vi "Process Data.vi"(8 "error in (no error)":errorcluster, 9 "Channel Data":T3 {"Current Values"."State" items=["Channel is stopped", "Channel is running", "Channel is paused"]; "Current Values"."I Range" items=["I range 100 pA SP-300 series", "I range 1 nA VMP3 / SP-300 series", "I range 10 nA VMP3 / SP-300 series", "I range 100 nA VMP3 / SP-300 series", "I range 1 uA VMP3 / SP-300 series", "I range 10 uA VMP3 / SP-300 series", "I range 100 uA VMP3 / SP-300 series", "I range 1 mA VMP3 / SP-300 series", "I range 10 mA VMP3 / SP-300 series", "I range 100 mA VMP3 / SP-300 series", "I range 1 A VMP3 / SP-300 series", "Booster VMP3 / SP-300 series", "Auto range VMP3 / SP-300 series"]; "Current Values"."Hardware Option Error Code" items=["No Error"=0, "no instrument connected"=-1, "connection in progress"=-2, "selected channel(s) unplugged"=-3, "invalid function parameters"=-4, "selected file does not exist"=-5, "function failed"=-6, "no channel selected"=-7, "invalid instrument configuration"=-8, "EC-Lab firmware loaded on the instrument"=-9, "library not correctly loaded in memory"=-10, "USB library not correctly loaded in memory"=-11, "function of the library already in progress"=-12, "selected channel(s) already used"=-13, "device not allowed"=-14, "Invalid update function parameters"=-15, "internal instrument communication failed"=-101, "too many data to transfer from the instrument (device error)"=-102, "selected channel(s) unplugged (device error)"=-103, "instrument response error"=-104, "invalid message size"=-105]}, 11 "Potentiostat Galvanostat in":refnum<class "Potentiostat Galvanostat.lvclass">) -> (0 "error out":errorcluster, 1 "Processed Data":T1, 2 "Column Names":T2, 3 "Potentiostat Galvanostat out":refnum<class "Potentiostat Galvanostat.lvclass">)   [LabVIEW 2018, in "Potentiostat Galvanostat.lvclass"]
uses:
  Potentiostat Galvanostat.lvclass
  Controls/Channel Data.ctl
  Controls/Process Data.ctl
  Controls/Data Information.ctl
  Controls/Technique ID.ctl
  Controls/Current Values.ctl
  Controls/Channel State.ctl
  Controls/Current Range.ctl
  Controls/Error Codes.ctl
  Controls/Processed Data Column Names.ctl
  Controls/Processed Data.ctl
  Potentiostat Galvanostat.lvclass/Potentiostat Galvanostat.ctl
  Controls/OCV Processed Data Columns.ctl
  Controls/CA-CP Processed Data Columns.ctl
  Controls/CV Processed Data Columns.ctl
  Controls/PEIS-GEIS P0 Processed Data Columns.ctl
  Controls/PEIS-GEIS P1 Processed Data Columns.ctl
  BL_GetErrorMsg.vi
  <vilib>/Utility/error.llb/Error Cluster From Error Code.vi
  <vilib>/Utility/Data Type/NI_Data Type.lvlib
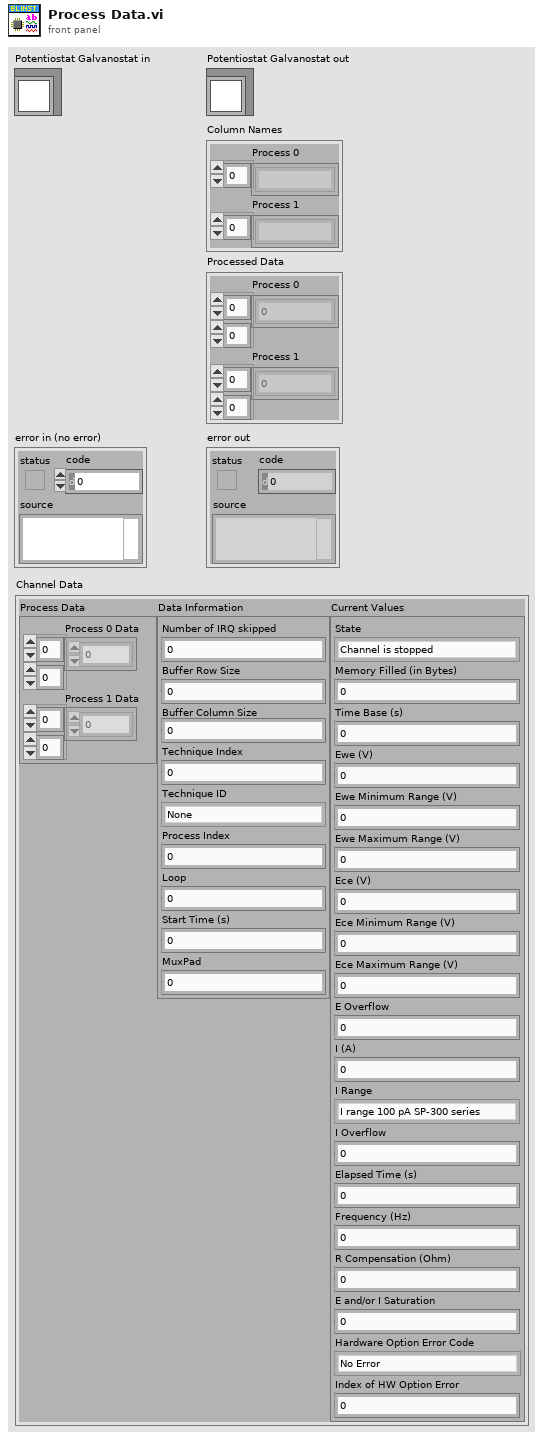
[diagram p1: front panel]
types:
  T1 = typedef "Potentiostat Galvanostat.lvclass/Processed Data.ctl" = cluster{"Process 0":dbl[][], "Process 1":dbl[][]}
  T2 = typedef "Potentiostat Galvanostat.lvclass/Processed Data Column Names.ctl" = cluster{"Process 0":string[], "Process 1":string[]}
  T3 = typedef "Potentiostat Galvanostat.lvclass/Channel Data.ctl" = cluster{"Process Data":T4, "Data Information":T5, "Current Values":T7}
  T4 = typedef "Potentiostat Galvanostat.lvclass/Process Data.ctl" = cluster{"Process 0 Data":sgl[][], "Process 1 Data":sgl[][]}
  T5 = typedef "Potentiostat Galvanostat.lvclass/Data Information.ctl" = cluster{"Number of IRQ skipped":i32, "Buffer Row Size":i32, "Buffer Column Size":i32, "Technique Index":i32, "Technique ID":T6, "Process Index":i32, "Loop":i32, "Start Time (s)":sgl, "MuxPad":i32}
  T6 = typedef "Potentiostat Galvanostat.lvclass/Technique ID.ctl" = i32
  T7 = typedef "Potentiostat Galvanostat.lvclass/Current Values.ctl" = cluster{"State":T8, "Memory Filled (in Bytes)":i32, "Time Base (s)":sgl, "Ewe (V)":sgl, "Ewe Minimum Range (V)":sgl, "Ewe Maximum Range (V)":sgl, "Ece (V)":sgl, "Ece Minimum Range (V)":sgl, "Ece Maximum Range (V)":sgl, "E Overflow":i32, "I (A)":sgl, "I Range":T9, "I Overflow":i32, "Elapsed Time (s)":dbl, "Frequency (Hz)":sgl, "R Compensation (Ohm)":sgl, "E and/or I Saturation":sgl, "Hardware Option Error Code":T10, "Index of HW Option Error":i32}
  T8 = typedef "Potentiostat Galvanostat.lvclass/Channel State.ctl" = i32
  T9 = typedef "Potentiostat Galvanostat.lvclass/Current Range.ctl" = i32
  T10 = typedef "Potentiostat Galvanostat.lvclass/Error Codes.ctl" = i32
  T11 = typedef "Potentiostat Galvanostat.lvclass/OCV Processed Data Columns.ctl" = enum16{"Time /s", "Ewe /V", "Ece /V"}
  T12 = typedef "Potentiostat Galvanostat.lvclass/CA-CP Processed Data Columns.ctl" = enum16{"Time /s", "Ewe /V", "I /A", "Cycle", "Q /C", "log(| I /A |)", "Power /W", "| Power /W |"}
  T13 = typedef "Potentiostat Galvanostat.lvclass/CV Processed Data Columns.ctl" = enum16{"Time /s", "Ece /V", "I /A", "Ewe /V", "Cycle", "Q /C", "log(| I /A |)", "Power /W", "| Power /W |"}
  T14 = typedef "Potentiostat Galvanostat.lvclass/PEIS-GEIS P0 Processed Data Columns.ctl" = enum16{"Time /s", "Ewe /V", "Iwe /A"}
  T15 = typedef "Potentiostat Galvanostat.lvclass/PEIS-GEIS P1 Processed Data Columns.ctl" = enum16{"Frequency /Hz", "| Ewe /V |", "| Iwe /A |", "Phase(Zwe) /rad", "Ewe /V", "Iwe /A", "Ewe Range", "| Ece /V |", "| Ice /A |", "Phase(Zce) /rad", "Ece /V", "Ice /A", "Ece Range", "Time /s", "I Range", "log(| Frequuency /Hz |)", "log(| Iwe /A |)", "log(| Ice /A  |)", "Phase(Zwe) /deg", "Phase(Zce) /deg", "Zwe /ohms", "Zce /ohms", "log(| Zwe /Ohms |)", "log(| Zce /Ohms |)", "-Im(Zwe) ", "-Im(Zce)", "Re(Zwe)", "Re(Zce)"}
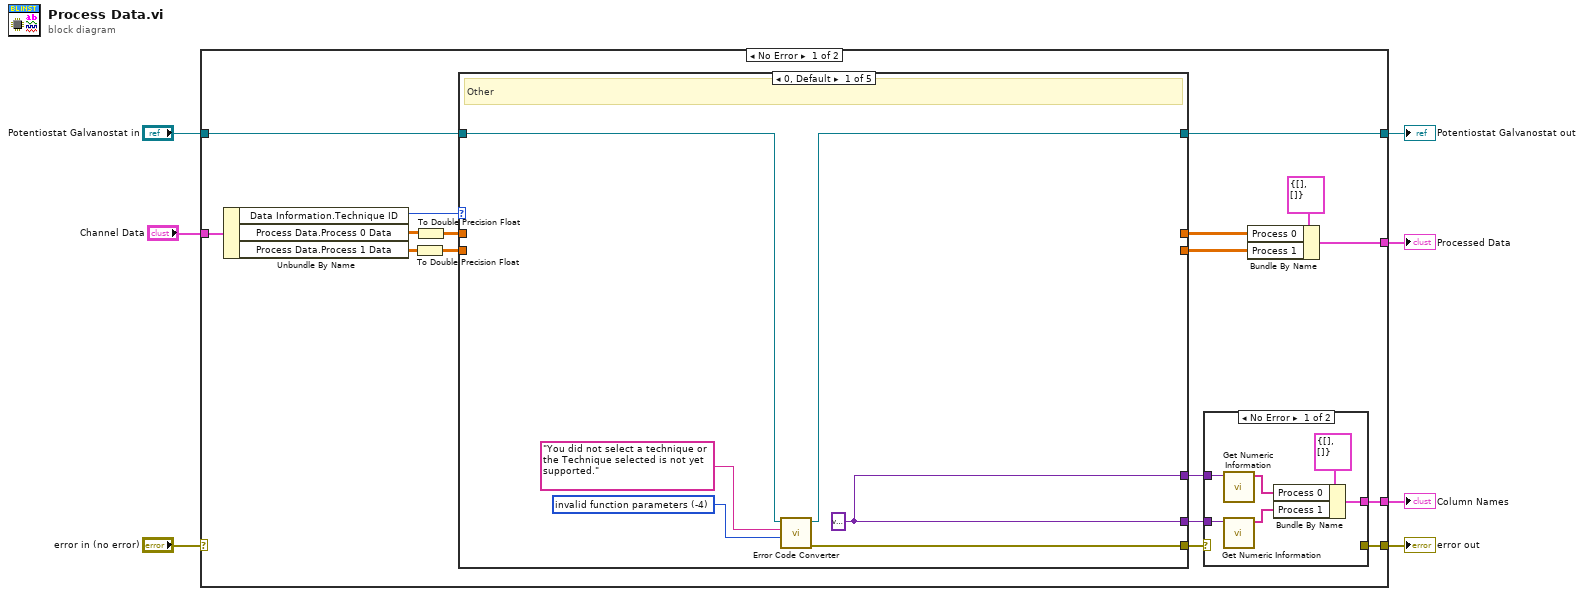
[diagram p0: block diagram]
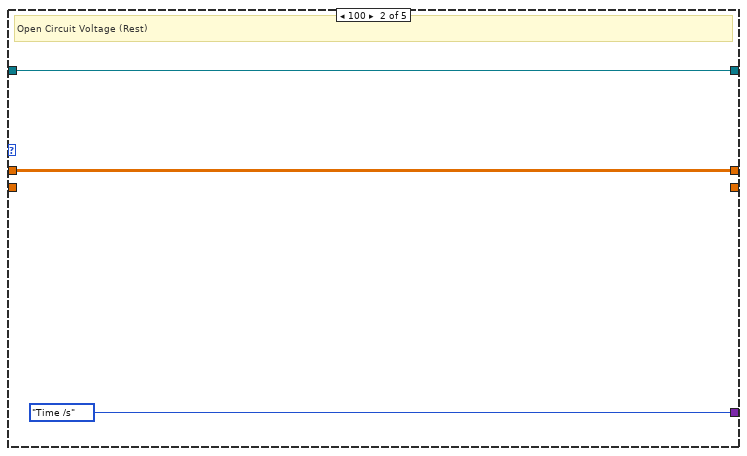
[diagram p3: hidden frame]
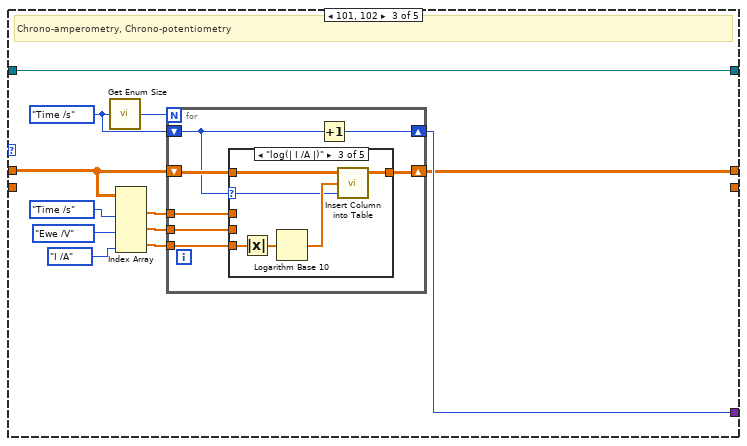
[diagram p4: hidden frame]
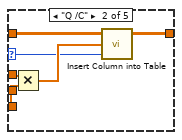
[diagram p6: hidden frame]
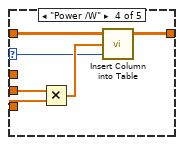
[diagram p7: hidden frame]
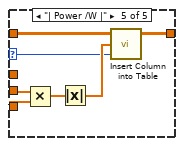
[diagram p8: hidden frame]
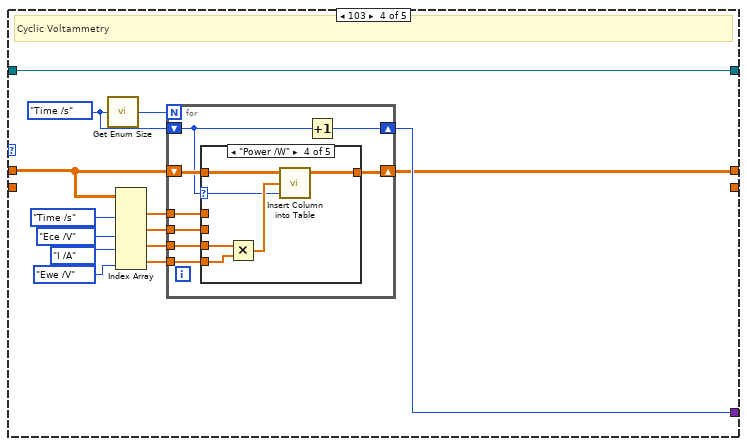
[diagram p9: hidden frame]
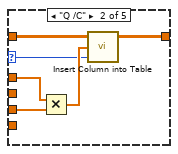
[diagram p11: hidden frame]
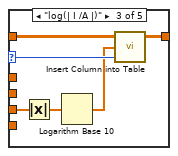
[diagram p12: hidden frame]
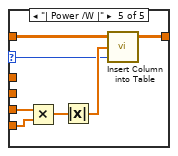
[diagram p13: hidden frame]
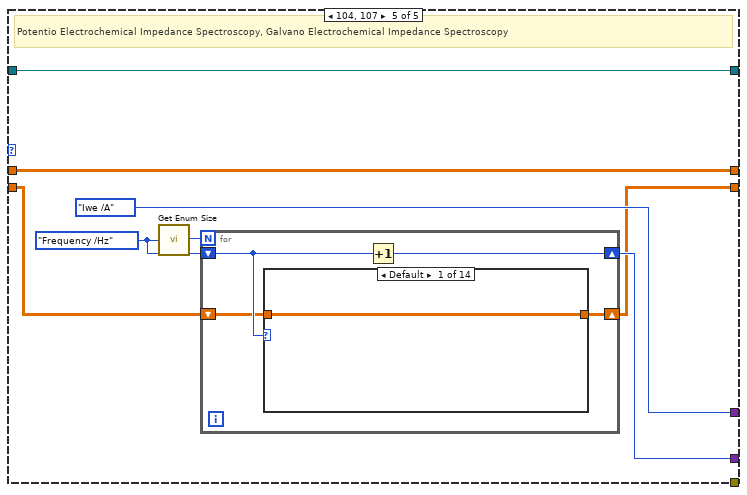
[diagram p14: hidden frame]
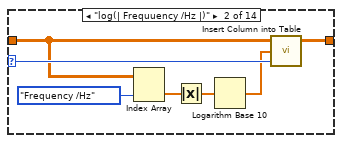
[diagram p15: hidden frame]
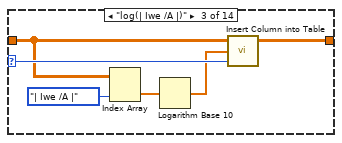
[diagram p16: hidden frame]
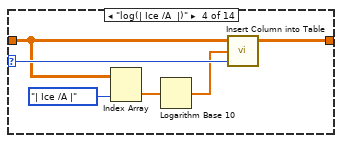
[diagram p17: hidden frame]
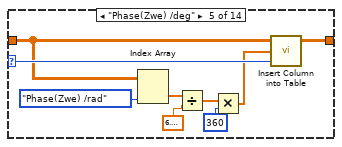
[diagram p18: hidden frame]
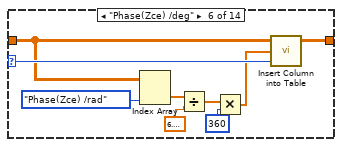
[diagram p19: hidden frame]
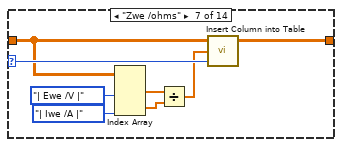
[diagram p20: hidden frame]
diagram:
  n1 = case shown="No Error" "error in (no error)" {
    selector: "error in (no error)" -> [_ w251]
    tunnel: "Channel Data" -> [w23 _]
    tunnel: [w20 w251] -> w6
    tunnel: "Potentiostat Galvanostat in" -> [w16 w250]
    tunnel: [w15 w250] -> w4
    tunnel: [w12 _] -> w2
    tunnel: [w8 _] -> w1
    frame No Error {
      n2 = Unbundle By Name(w23) -> ("Data Information.Technique ID"=w24:T6, "Process Data.Process 0 Data"=w18:sgl[][], "Process Data.Process 1 Data"=w17:sgl[][])
      n3 = To Double Precision Float(number=w17) -> (double precision float=w21:dbl[][])
      n4 = To Double Precision Float(number=w18) -> (double precision float=w22:dbl[][])
      n5 = case shown="0, Default" w24 {
        tunnel: w22 -> [_ w38 w44 w89 w135]
        tunnel: w21 -> [_ _ _ _ w139]
        tunnel: [w36 _ _ _ _] -> w14
        tunnel: [w32 _ _ _ w141] -> w19
        tunnel: w16 -> [w34 w40 w43 w88 w137]
        tunnel: [w35 w40 w43 w88 w137] -> w15
        tunnel: [w32 OCV_Processed_Data_Columns."Time /s" w42 w87 PEIS-GEIS_P0_Processed_Data_Columns."Iwe /A" ("Enum")] -> w13
        tunnel: [_ w38 w41 w86 w135] -> w10
        tunnel: [_ _ _ _ w134] -> w9
        frame 0, Default {
          w37 = T10 -4 items=["No Error"=0, "no instrument connected"=-1, "connection in progress"=-2, "selected channel(s) unplugged"=-3, "invalid function parameters"=-4, "selected file does not exist"=-5, "function failed"=-6, "no channel selected"=-7, "invalid instrument configuration"=-8, "EC-Lab firmware loaded on the instrument"=-9, "library not correctly loaded in memory"=-10, "USB library not correctly loaded in memory"=-11, "function of the library already in progress"=-12, "selected channel(s) already used"=-13, "device not allowed"=-14, "Invalid update function parameters"=-15, "internal instrument communication failed"=-101, "too many data to transfer from the instrument (device error)"=-102, "selected channel(s) unplugged (device error)"=-103, "instrument response error"=-104, "invalid message size"=-105] ("Error Code")
          w32 = variant
          # "Other"
          n6 = call "Error Code Converter.vi"("Error Code"=w37, "Additional Description"="You did not select a technique or the Technique selected is not yet supported.", "Potentiostat Galvanostat in"=w34) -> ("error out"=w36:errorcluster, "Potentiostat Galvanostat out"=w35:refnum<class "Potentiostat Galvanostat.lvclass">)  [unwired: 7 in]
        }
        frame 100 {
          # "Open Circuit Voltage (Rest)"
        }
        frame 101, 102 {
          w45 = CA-CP_Processed_Data_Columns."Time /s"
          # "Chrono-amperometry, Chrono-potentiometry"
          n7 = call "Get Enum Size.vi"("Enum"=w45) -> ("Size"=w46:i32)  [unwired: 4 in]
          n8 = Index Array(array=w44, index (col) #1=CA-CP_Processed_Data_Columns."Time /s", index (col) #2=CA-CP_Processed_Data_Columns."Ewe /V", index (col) #3=CA-CP_Processed_Data_Columns."I /A") -> (element #1=w50:dbl[], element #2=w51:dbl[], element #3=w52:dbl[])  [unwired: 3 in]
          n9 = for {
            N: w46 -> [_]
            tunnel: w52 -> [w56]
            tunnel: w51 -> [w57]
            tunnel: w50 -> [w58]
            shift-right: [w59] -> w41
            shift-left: w44 -> [w55]
            shift-right: [w53] -> w42
            shift-left: w45 -> [w54]
            n10 = case shown="\"log(| I /A |)\"" w54 {
              selector: w54 -> [_ w61 w67 w73 w79]
              tunnel: [w60 w66 w72 w76 w84] -> w59
              tunnel: w55 -> [w60 w65 w71 w75 w85]
              tunnel: w58 -> [_ w63 _ _ _]
              tunnel: w57 -> [_ _ _ w78 w83]
              tunnel: w56 -> [_ w64 w70 w77 w82]
              frame Default {
              }
              frame "Q /C" {
                # "Q /C"
                n11 = Multiply(x=w63, y=w64) -> (x*y=w62:dbl[])
                n12 = call "Insert Column into Table.vi"("Index"=w61, "Column in"=w62, "Table in"=w65) -> ("Table out"=w66:dbl[][])  [unwired: 2 in]
              }
              frame "log(| I /A |)" {
                # "log(| I /A |)"
                n13 = Absolute Value(x=w70) -> (abs(x)=w69:dbl[])
                n14 = Logarithm Base 10(1:w69) -> (0:w68:dbl[])
                n15 = call "Insert Column into Table.vi"("Index"=w67, "Column in"=w68, "Table in"=w71) -> ("Table out"=w72:dbl[][])  [unwired: 2 in]
              }
              frame "Power /W" {
                # "Power /W"
                n16 = Multiply(x=w78, y=w77) -> (x*y=w74:dbl[])
                n17 = call "Insert Column into Table.vi"("Index"=w73, "Column in"=w74, "Table in"=w75) -> ("Table out"=w76:dbl[][])  [unwired: 2 in]
              }
              frame "| Power /W |" {
                # "| Power /W|"
                n18 = Multiply(x=w83, y=w82) -> (x*y=w81:dbl[])
                n19 = Absolute Value(x=w81) -> (abs(x)=w80:dbl[])
                n20 = call "Insert Column into Table.vi"("Index"=w79, "Column in"=w80, "Table in"=w85) -> ("Table out"=w84:dbl[][])  [unwired: 2 in]
              }
            }
            n21 = Increment(x=w54) -> (x+1=w53:T12)
          }
        }
        frame 103 {
          w90 = CV_Processed_Data_Columns."Time /s"
          # "Cyclic Voltammetry"
          n22 = call "Get Enum Size.vi"("Enum"=w90) -> ("Size"=w91:i32)  [unwired: 4 in]
          n23 = Index Array(array=w89, index (col) #1=CV_Processed_Data_Columns."Time /s", index (col) #2=CV_Processed_Data_Columns."Ece /V", index (col) #3=CV_Processed_Data_Columns."I /A", index (col) #4=CV_Processed_Data_Columns."Ewe /V") -> (element #1=w97:dbl[], element #2=w98:dbl[], element #3=w99:dbl[], element #4=w96:dbl[])  [unwired: 4 in]
          n24 = for {
            N: w91 -> [_]
            tunnel: w99 -> [w103]
            tunnel: w98 -> [w104]
            tunnel: w97 -> [w105]
            shift-right: [w107] -> w86
            shift-left: w89 -> [w106]
            tunnel: w96 -> [w102]
            shift-right: [w100] -> w87
            shift-left: w90 -> [w101]
            n25 = case shown="\"Power /W\"" w101 {
              selector: w101 -> [_ w109 w116 w121 w127]
              tunnel: [w108 w114 w120 w126 w133] -> w107
              tunnel: w106 -> [w108 w110 w117 w122 w128]
              tunnel: w105 -> [_ w112 _ _ _]
              tunnel: w104 -> [_ _ _ _ _]
              tunnel: w103 -> [_ w113 w119 w124 w129]
              tunnel: w102 -> [_ _ _ w123 w130]
              frame Default {
              }
              frame "Q /C" {
                # "Q /C"
                n26 = Multiply(x=w112, y=w113) -> (x*y=w111:dbl[])
                n27 = call "Insert Column into Table.vi"("Index"=w109, "Column in"=w111, "Table in"=w110) -> ("Table out"=w114:dbl[][])  [unwired: 2 in]
              }
              frame "log(| I /A |)" {
                # "log(| I /A |)"
                n28 = Absolute Value(x=w119) -> (abs(x)=w118:dbl[])
                n29 = Logarithm Base 10(1:w118) -> (0:w115:dbl[])
                n30 = call "Insert Column into Table.vi"("Index"=w116, "Column in"=w115, "Table in"=w117) -> ("Table out"=w120:dbl[][])  [unwired: 2 in]
              }
              frame "Power /W" {
                # "Power /W"
                n31 = Multiply(x=w124, y=w123) -> (x*y=w125:dbl[])
                n32 = call "Insert Column into Table.vi"("Index"=w121, "Column in"=w125, "Table in"=w122) -> ("Table out"=w126:dbl[][])  [unwired: 2 in]
              }
              frame "| Power /W |" {
                # "| Power /W|"
                n33 = Multiply(x=w129, y=w130) -> (x*y=w132:dbl[])
                n34 = Absolute Value(x=w132) -> (abs(x)=w131:dbl[])
                n35 = call "Insert Column into Table.vi"("Index"=w127, "Column in"=w131, "Table in"=w128) -> ("Table out"=w133:dbl[][])  [unwired: 2 in]
              }
            }
            n36 = Increment(x=w101) -> (x+1=w100:T13)
          }
        }
        frame 104, 107 {
          w140 = PEIS-GEIS_P1_Processed_Data_Columns."Frequency /Hz" ("PEIS")
          # "Potentio Electrochemical Impedance Spectroscopy, Galvano Electrochemical Impedance Spectroscopy"
          n37 = call "Get Enum Size.vi"("Enum"=w140) -> ("Size"=w138:i32)  [unwired: 4 in]
          n38 = for {
            N: w138 -> [_]
            shift-right: [w145] -> w141
            shift-left: w140 -> [w144]
            shift-right: [w143] -> w134
            shift-left: w139 -> [w142]
            n39 = case shown="Default" w144 {
              selector: w144 -> [_ w152 w158 w164 w173 w182 w190 w198 w204 w210 w220 w230 w239 w248]
              tunnel: [w146 w153 w159 w165 w174 w183 w191 w199 w205 w211 w221 w231 w240 w249] -> w143
              tunnel: w142 -> [w146 w151 w157 w163 w172 w181 w189 w197 w203 w209 w219 w229 w238 w247]
              frame Default {
              }
              frame "log(| Frequuency /Hz |)" {
                n40 = Index Array(array=w151, index (col)=PEIS-GEIS_P1_Processed_Data_Columns."Frequency /Hz" ("PEIS")) -> (element=w149:dbl[])  [unwired: 1 in]
                n41 = Absolute Value(x=w149) -> (abs(x)=w148:dbl[])
                n42 = Logarithm Base 10(1:w148) -> (0:w147:dbl[])
                n43 = call "Insert Column into Table.vi"("Index"=w152, "Column in"=w147, "Table in"=w151) -> ("Table out"=w153:dbl[][])  [unwired: 2 in]
              }
              frame "log(| Iwe /A |)" {
                n44 = Index Array(array=w157, index (col)=PEIS-GEIS_P1_Processed_Data_Columns."| Iwe /A |" ("PEIS")) -> (element=w154:dbl[])  [unwired: 1 in]
                n45 = Logarithm Base 10(1:w154) -> (0:w155:dbl[])
                n46 = call "Insert Column into Table.vi"("Index"=w158, "Column in"=w155, "Table in"=w157) -> ("Table out"=w159:dbl[][])  [unwired: 2 in]
              }
              frame "log(| Ice /A  |)" {
                n47 = Index Array(array=w163, index (col)=PEIS-GEIS_P1_Processed_Data_Columns."| Ice /A |" ("PEIS")) -> (element=w160:dbl[])  [unwired: 1 in]
                n48 = Logarithm Base 10(1:w160) -> (0:w161:dbl[])
                n49 = call "Insert Column into Table.vi"("Index"=w164, "Column in"=w161, "Table in"=w163) -> ("Table out"=w165:dbl[][])  [unwired: 2 in]
              }
              frame "Phase(Zwe) /deg" {
                n50 = Index Array(array=w172, index (col)=PEIS-GEIS_P1_Processed_Data_Columns."Phase(Zwe) /rad" ("PEIS")) -> (element=w167:dbl[])  [unwired: 1 in]
                n51 = Divide(x=w167, y=6.283185307179586) -> (x/y=w169:dbl[])
                n52 = Multiply(x=w169, y=360) -> (x*y=w166:dbl[])
                n53 = call "Insert Column into Table.vi"("Index"=w173, "Column in"=w166, "Table in"=w172) -> ("Table out"=w174:dbl[][])  [unwired: 2 in]
              }
              frame "Phase(Zce) /deg" {
                n54 = Index Array(array=w181, index (col)=PEIS-GEIS_P1_Processed_Data_Columns."Phase(Zce) /rad" ("PEIS")) -> (element=w176:dbl[])  [unwired: 1 in]
                n55 = Divide(x=w176, y=6.283185307179586) -> (x/y=w178:dbl[])
                n56 = Multiply(x=w178, y=360) -> (x*y=w175:dbl[])
                n57 = call "Insert Column into Table.vi"("Index"=w182, "Column in"=w175, "Table in"=w181) -> ("Table out"=w183:dbl[][])  [unwired: 2 in]
              }
              frame "Zwe /ohms" {
                n58 = Index Array(array=w189, index (col) #1=PEIS-GEIS_P1_Processed_Data_Columns."| Ewe /V |" ("PEIS"), index (col) #2=PEIS-GEIS_P1_Processed_Data_Columns."| Iwe /A |" ("PEIS")) -> (element #1=w187:dbl[], element #2=w185:dbl[])  [unwired: 2 in]
                n59 = Divide(x=w187, y=w185) -> (x/y=w186:dbl[])
                n60 = call "Insert Column into Table.vi"("Index"=w190, "Column in"=w186, "Table in"=w189) -> ("Table out"=w191:dbl[][])  [unwired: 2 in]
              }
              frame "Zce /ohms" {
                n61 = Index Array(array=w197, index (col) #1=PEIS-GEIS_P1_Processed_Data_Columns."| Ece /V |" ("PEIS"), index (col) #2=PEIS-GEIS_P1_Processed_Data_Columns."| Ice /A |" ("PEIS")) -> (element #1=w195:dbl[], element #2=w193:dbl[])  [unwired: 2 in]
                n62 = Divide(x=w195, y=w193) -> (x/y=w194:dbl[])
                n63 = call "Insert Column into Table.vi"("Index"=w198, "Column in"=w194, "Table in"=w197) -> ("Table out"=w199:dbl[][])  [unwired: 2 in]
              }
              frame "log(| Zwe /Ohms |)" {
                n64 = Index Array(array=w203, index (col)=PEIS-GEIS_P1_Processed_Data_Columns."Zwe /ohms" ("PEIS")) -> (element=w201:dbl[])  [unwired: 1 in]
                n65 = Logarithm Base 10(1:w201) -> (0:w200:dbl[])
                n66 = call "Insert Column into Table.vi"("Index"=w204, "Column in"=w200, "Table in"=w203) -> ("Table out"=w205:dbl[][])  [unwired: 2 in]
              }
              frame "log(| Zce /Ohms |)" {
                n67 = Index Array(array=w209, index (col)=PEIS-GEIS_P1_Processed_Data_Columns."Zce /ohms" ("PEIS")) -> (element=w207:dbl[])  [unwired: 1 in]
                n68 = Logarithm Base 10(1:w207) -> (0:w206:dbl[])
                n69 = call "Insert Column into Table.vi"("Index"=w210, "Column in"=w206, "Table in"=w209) -> ("Table out"=w211:dbl[][])  [unwired: 2 in]
              }
              frame "-Im(Zwe) " {
                n70 = Index Array(array=w219, index (col) #1=PEIS-GEIS_P1_Processed_Data_Columns."Zwe /ohms" ("PEIS"), index (col) #2=PEIS-GEIS_P1_Processed_Data_Columns."Phase(Zwe) /rad" ("PEIS")) -> (element #1=w214:dbl[], element #2=w213:dbl[])  [unwired: 2 in]
                n71 = Sine(x=w213) -> (sin(x)=w216:dbl[])
                n72 = Compound Arithmetic op=MULTIPLY(-1.0, w214, w216) -> (w212:dbl[])
                n73 = call "Insert Column into Table.vi"("Index"=w220, "Column in"=w212, "Table in"=w219) -> ("Table out"=w221:dbl[][])  [unwired: 2 in]
              }
              frame "-Im(Zce)" {
                n74 = Index Array(array=w229, index (col) #1=PEIS-GEIS_P1_Processed_Data_Columns."Zce /ohms" ("PEIS"), index (col) #2=PEIS-GEIS_P1_Processed_Data_Columns."Phase(Zce) /rad" ("PEIS")) -> (element #1=w225:dbl[], element #2=w227:dbl[])  [unwired: 2 in]
                n75 = Sine(x=w227) -> (sin(x)=w223:dbl[])
                n76 = Compound Arithmetic op=MULTIPLY(-1.0, w225, w223) -> (w224:dbl[])
                n77 = call "Insert Column into Table.vi"("Index"=w230, "Column in"=w224, "Table in"=w229) -> ("Table out"=w231:dbl[][])  [unwired: 2 in]
              }
              frame "Re(Zwe)" {
                n78 = Index Array(array=w238, index (col) #1=PEIS-GEIS_P1_Processed_Data_Columns."Zwe /ohms" ("PEIS"), index (col) #2=PEIS-GEIS_P1_Processed_Data_Columns."Phase(Zwe) /rad" ("PEIS")) -> (element #1=w236:dbl[], element #2=w235:dbl[])  [unwired: 2 in]
                n79 = Cosine(x=w235) -> (cos(x)=w234:dbl[])
                n80 = Multiply(x=w236, y=w234) -> (x*y=w232:dbl[])
                n81 = call "Insert Column into Table.vi"("Index"=w239, "Column in"=w232, "Table in"=w238) -> ("Table out"=w240:dbl[][])  [unwired: 2 in]
              }
              frame "Re(Zce)" {
                n82 = Index Array(array=w247, index (col) #1=PEIS-GEIS_P1_Processed_Data_Columns."Zce /ohms" ("PEIS"), index (col) #2=PEIS-GEIS_P1_Processed_Data_Columns."Phase(Zce) /rad" ("PEIS")) -> (element #1=w245:dbl[], element #2=w244:dbl[])  [unwired: 2 in]
                n83 = Cosine(x=w244) -> (cos(x)=w243:dbl[])
                n84 = Multiply(x=w245, y=w243) -> (x*y=w241:dbl[])
                n85 = call "Insert Column into Table.vi"("Index"=w248, "Column in"=w241, "Table in"=w247) -> ("Table out"=w249:dbl[][])  [unwired: 2 in]
              }
            }
            n86 = Increment(x=w144) -> (x+1=w145:T15)
          }
        }
      }
      n87 = case shown="No Error" w14 {
        selector: w14 -> [_ w31]
        tunnel: [_ w31] -> w20
        tunnel: w19 -> [w30 _]
        tunnel: w13 -> [w29 _]
        tunnel: [w25 _] -> w12
        frame No Error {
          n88 = call <vilib>:"Get Numeric Information.vi"("Variant"=w29) -> ("Enum Names"=w26:string[])  [unwired: 7 in, 3 out]
          n89 = call <vilib>:"Get Numeric Information.vi"("Variant"=w30) -> ("Enum Names"=w27:string[])  [unwired: 7 in, 3 out]
          n90 = Bundle By Name(cluster=T2 {"Process 0"=[], "Process 1"=[]} ("Column Names"), "Process 0"=w26, "Process 1"=w27) -> (w25:T2)
        }
        frame Error {
        }
      }
      n91 = Bundle By Name(cluster=T1 {"Process 0"=[], "Process 1"=[]} ("Processed Data"), "Process 0"=w10, "Process 1"=w9) -> (w8:T1)
    }
    frame Error {
    }
  }
  "error out" <- w6
  "Potentiostat Galvanostat out" <- w4
  "Column Names" <- w2
  "Processed Data" <- w1
